vi "Get f0.vi"(8 "error in":errorcluster, 11 "PAS Data in":refnum<class "PAS Data.lvclass">) -> (0 "error out":errorcluster, 2 "f0":sgl, 3 "PAS Data out":refnum<class "PAS Data.lvclass">)   [LabVIEW 2014, in "PAS Library.lvlib" / "PAS Data.lvclass"]
uses:
  PAS Data.lvclass
  PAS Data.lvclass/PAS Data.ctl
  Cell/PAS Cell Data.lvclass
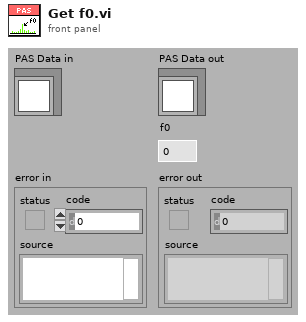
[diagram p1: front panel]
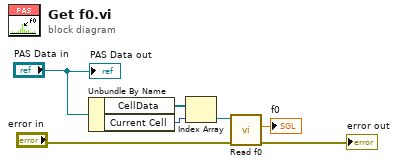
[diagram p0: block diagram]
diagram:
  n1 = Unbundle By Name("PAS Data in") -> ("CellData"=w6:refnum<class "PAS Cell Data.lvclass">[], "Current Cell"=w5:i32)
  n2 = Index Array(array=w6, index=w5) -> (element=w4:refnum<class "PAS Cell Data.lvclass">)
  n3 = call "Read f0.vi"("error in (no error)"="error in", "PAS Cell Data in"=w4) -> ("error out"=→"error out":errorcluster, "f0"=→"f0":sgl)  [unwired: 7 in, 1 out]
  "PAS Data out" <- "PAS Data in"
